vi "set_pixel_frequency.vi"(8 "error in (no error)":errorcluster, 10 "pixel frequency":dbl[unit], 11 "FPGAWrapperMH120124FrameScan_PXI7813R in":refnum<class "FPGAWrapperMH120124FrameScan_PXI7813R.lvclass">) -> (0 "error out":errorcluster, 3 "FPGAWrapperMH120124FrameScan_PXI7813R out":refnum<class "FPGAWrapperMH120124FrameScan_PXI7813R.lvclass">)   [LabVIEW 2010, in "FPGAWrapperMH120124FrameScan_PXI7813R.lvclass"]
uses:
  FPGAWrapperMH120124FrameScan_PXI7813R.lvclass
  FPGAWrapperMH120124FrameScan_PXI7813R.lvclass/FPGAWrapperMH120124FrameScan_PXI7813R.ctl
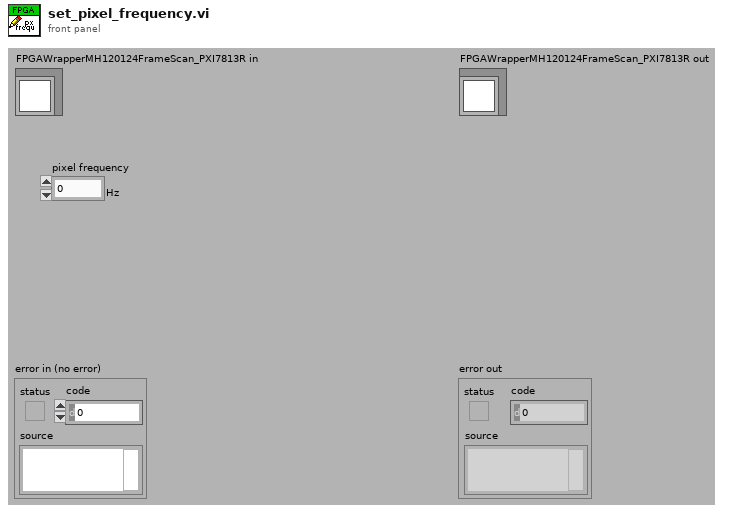
[diagram p1: front panel]
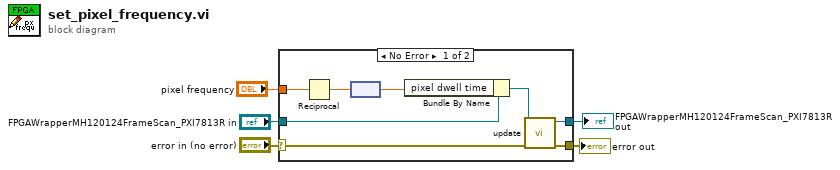
[diagram p0: block diagram]
diagram:
  n1 = case shown="No Error" "error in (no error)" {
    selector: "error in (no error)" -> [w12 w15]
    tunnel: [w8 w15] -> w5
    tunnel: "pixel frequency" -> [w11 _]
    tunnel: "FPGAWrapperMH120124FrameScan_PXI7813R in" -> [w7 w14]
    tunnel: [w6 w14] -> w1
    frame No Error {
      n2 = Reciprocal(x=w11) -> (1/x=w10:dbl[unit])
      n3 = node(w10) -> (w9:dbl)
      n4 = Bundle By Name(cluster=w7, "pixel dwell time"=w9) -> (w13:refnum<class "FPGAWrapperMH120124FrameScan_PXI7813R.lvclass">)
      n5 = call-dynamic "update.vi"("error in (no error)"=w12, "FPGAWrapperMH120124FrameScan_PXI7813R in"=w13) -> ("error out"=w8:errorcluster, "FPGAWrapperMH120124FrameScan_PXI7813R out"=w6:refnum<class "FPGAWrapperMH120124FrameScan_PXI7813R.lvclass">)  [unwired: 8 in]
    }
    frame Error {
    }
  }
  "error out" <- w5
  "FPGAWrapperMH120124FrameScan_PXI7813R out" <- w1
